vi "Find Closest Port.vi"(8 "error in (no error)":errorcluster, 10 "point":cluster{"x":i16, "y":i16}, 11 "FSM.Node in":refnum<class "FSM.Node.lvclass">) -> (0 "error out":errorcluster, 1 "Location":cluster{"x":i16, "y":i16}, 2 "Port":refnum<class "FSM.Port.lvclass">, 3 "FSM.Node out":refnum<class "FSM.Node.lvclass">)   [LabVIEW 2020, in "FSM.Node.lvclass"]
uses:
  FSM.Node.lvclass
  FSM.Port/FSM.Port.lvclass
  FSM.Node.lvclass/FSM.Node.ctl
  FSM.Port/FSM.Port.lvclass/FSM.Port.ctl
  FSM.Port/Read Location.vi
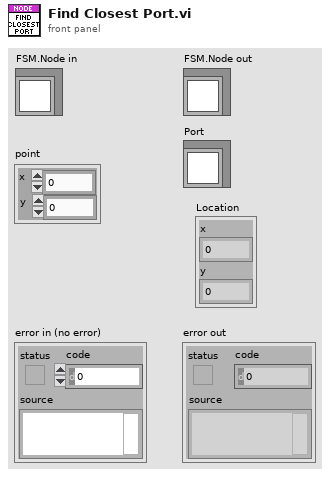
[diagram p1: front panel]
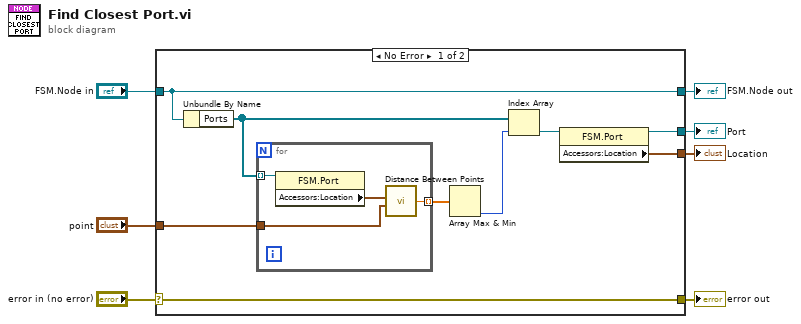
[diagram p0: block diagram]
diagram:
  n1 = case shown="No Error" "error in (no error)" {
    selector: "error in (no error)" -> [w16 w22]
    tunnel: [w16 w22] -> w6
    tunnel: [w15 w21] -> w4
    tunnel: "FSM.Node in" -> [w15 w21]
    tunnel: "point" -> [w14 _]
    tunnel: [w9 _] -> w2
    tunnel: [w8 _] -> w1
    frame No Error {
      n2 = Unbundle By Name(w15) -> ("Ports"=w12:refnum<class "FSM.Port.lvclass">[])
      n3 = for {
        tunnel: w12 -> [w20] mode=indexing
        tunnel: w14 -> [w18]
        tunnel: [w17] -> w13 mode=indexing
        n4 = property class="FSM.Port"(reference=w20) -> ("Accessors:Location"=w19:cluster{"x":i16, "y":i16})  [unwired: 1 in, 2 out]
        n5 = call "Distance Between Points.vi"("B"=w18, "A"=w19) -> ("distance"=w17:dbl)  [unwired: 4 in]
      }
      n6 = Array Max & Min(array=w13) -> (min index (indices)=w11:i32)  [unwired: 3 out]
      n7 = Index Array(array=w12, index=w11) -> (element=w10:refnum<class "FSM.Port.lvclass">)
      n8 = property class="FSM.Port"(reference=w10) -> (reference out=w9:refnum<class "FSM.Port.lvclass">, "Accessors:Location"=w8:cluster{"x":i16, "y":i16})  [unwired: 1 in, 1 out]
    }
    frame Error {
    }
  }
  "error out" <- w6
  "FSM.Node out" <- w4
  "Port" <- w2
  "Location" <- w1
